vi "Load Config.vi"(8 "error in":errorcluster, 10 "config":string="config.ini", 11 "base path":path) -> (0 "error out":errorcluster, 3 "?":T1)   [LabVIEW 2014]
uses:
  Config.ctl
  <vilib>/Utility/config.llb/Read Key (String).vi
  <vilib>/Utility/config.llb/NI_LVConfig.lvlib
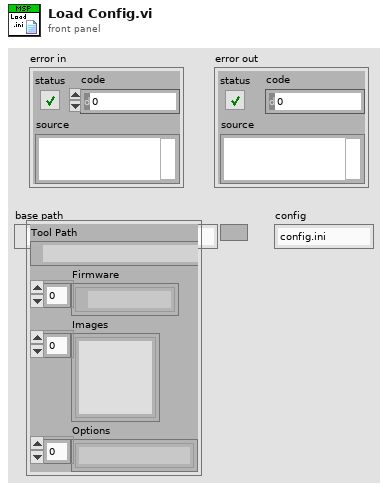
[diagram p1: front panel]
types:
  T1 = typedef "Config.ctl" = cluster{"Tool Path":path, "Firmware":path[], "Images":picture[], "Options":string[]}
  T2 = typedef "NI_LVConfig.lvlib/Config Data RefNum.ctl" = refnum<k1>
  T3 = typedef "imagedata.ctl" = cluster{"image type":i32, "image depth":i32, "image":u8[], "mask":u8[], "colors":u32[], "Rectangle":cluster{"left":i16, "top":i16, "right":i16, "bottom":i16}}
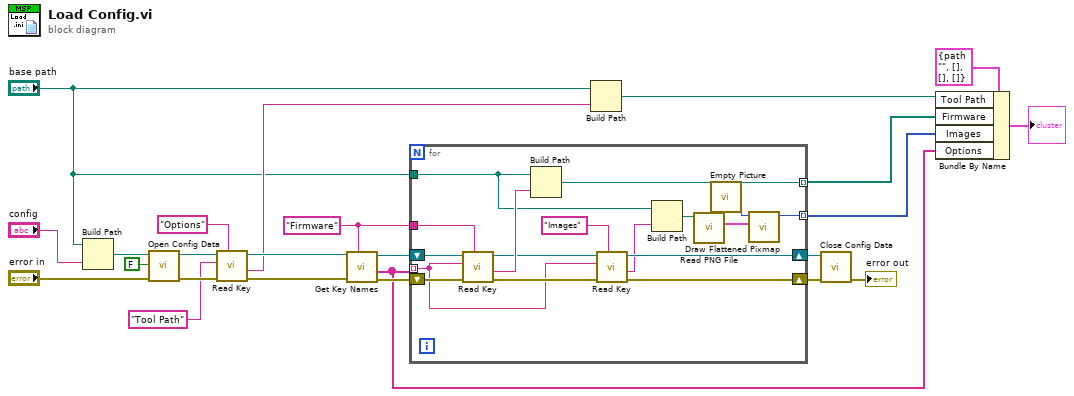
[diagram p0: block diagram]
diagram:
  w10 = "Firmware" ("section")
  n1 = Build Path(base path="base path", name or relative path="config") -> (appended path=w22:path)
  n2 = call <vilib>:"Open Config Data.vi"("error in (no error)"="error in", "create file if necessary (T)"=FALSE, "configuration file path"=w22) -> ("error out"=w24:errorcluster, "refnum"=w20:T2)  [unwired: 6 in, 1 out]
  n3 = call-poly <vilib>:"Read Key.vi"("section"="Options", "error in (no error)"=w24, "key"="Tool Path", "refnum"=w20) -> ("error out"=w17:errorcluster, "value"=w8:string, "refnum out"=w13:T2)  [unwired: 4 in, 1 out]
  n4 = call <vilib>:"Get Key Names.vi"("section"=w10, "error in (no error)"=w17, "refnum"=w13) -> ("error out"=w16:errorcluster, "key names"=w3:string[], "refnum out"=w12:T2)  [unwired: 5 in, 1 out]
  n5 = for {
    shift-right: [w35] -> w15
    shift-left: w16 -> [w41]
    shift-right: [w36] -> w11
    shift-left: w12 -> [w40]
    tunnel: w3 -> [w32] mode=indexing
    tunnel: w10 -> [w39]
    tunnel: "base path" -> [w30]
    tunnel: [w37] -> w4 mode=indexing
    tunnel: [w25] -> w1 mode=indexing
    n6 = call-poly <vilib>:"Read Key.vi"("section"=w39, "error in (no error)"=w41, "key"=w32, "refnum"=w40) -> ("error out"=w33:errorcluster, "value"=w38:string, "refnum out"=w34:T2)  [unwired: 4 in, 1 out]
    n7 = Build Path(base path=w30, name or relative path=w38) -> (appended path=w37:path)
    n8 = call-poly <vilib>:"Read Key.vi"("section"="Images", "error in (no error)"=w33, "key"=w32, "refnum"=w34) -> ("error out"=w35:errorcluster, "value"=w29:string, "refnum out"=w36:T2)  [unwired: 4 in, 1 out]
    n9 = Build Path(base path=w30, name or relative path=w29) -> (appended path=w28:path)
    n10 = call <vilib>:"Read PNG File.vi"("path to PNG file"=w28) -> ("image data"=w27:T3)  [unwired: 8 in, 2 out]
    n11 = call "Empty Picture"() -> ("empty picture"=w26:picture)
    n12 = call <vilib>:"Draw Flattened Pixmap.vi"("image data"=w27, "picture"=w26) -> ("new picture"=w25:picture)  [unwired: 7 in]
  }
  n13 = Build Path(base path="base path", name or relative path=w8) -> (appended path=w5:path)
  n14 = call <vilib>:"Close Config Data.vi"("error in (no error)"=w15, "refnum"=w11) -> ("error out"=→"error out":errorcluster)  [unwired: 8 in, 1 out]
  n15 = Bundle By Name(cluster=T1 {"Tool Path"=path "", "Firmware"=[], "Images"=[], "Options"=[]}, "Tool Path"=w5, "Firmware"=w4, "Images"=w1, "Options"=w3) -> (→"?":T1)
